vi "GetI.vi"(8 "error in (no error)":errorcluster, 11 "reference in":refnum<class "GOOP4_Sub.lvclass">) -> (0 "error out":errorcluster, 1 "Str 3":string, 2 "i 3":i32, 3 "reference in":refnum<class "GOOP4_Sub.lvclass">)   [LabVIEW 2019, in "GOOP4_Sub.lvclass"]
uses:
  GOOP4_Sub.lvclass
  GOOP4_Base_class/GOOP4_Base.lvclass
  C:/Users/Tiba/Desktop/1GOOP4_CreateObjects_Open_GDS/GOOP4_Base_class/GOOP4_Base.lvclass
panel:
  out "i 2":i32
  out "Str 2":string
  out "Str":string
  out "i":i32
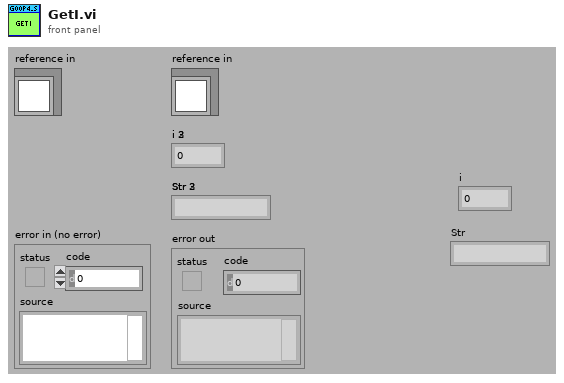
[diagram p1: front panel]
types:
  T1 = typedef "GOOP4_Sub.lvclass/ObjectAttributes.ctl" = cluster{"Str":string, "Boolean":bool}
  T2 = typedef "GOOP4_Base.lvclass/ObjectAttributes.ctl" = cluster{"i":i32}
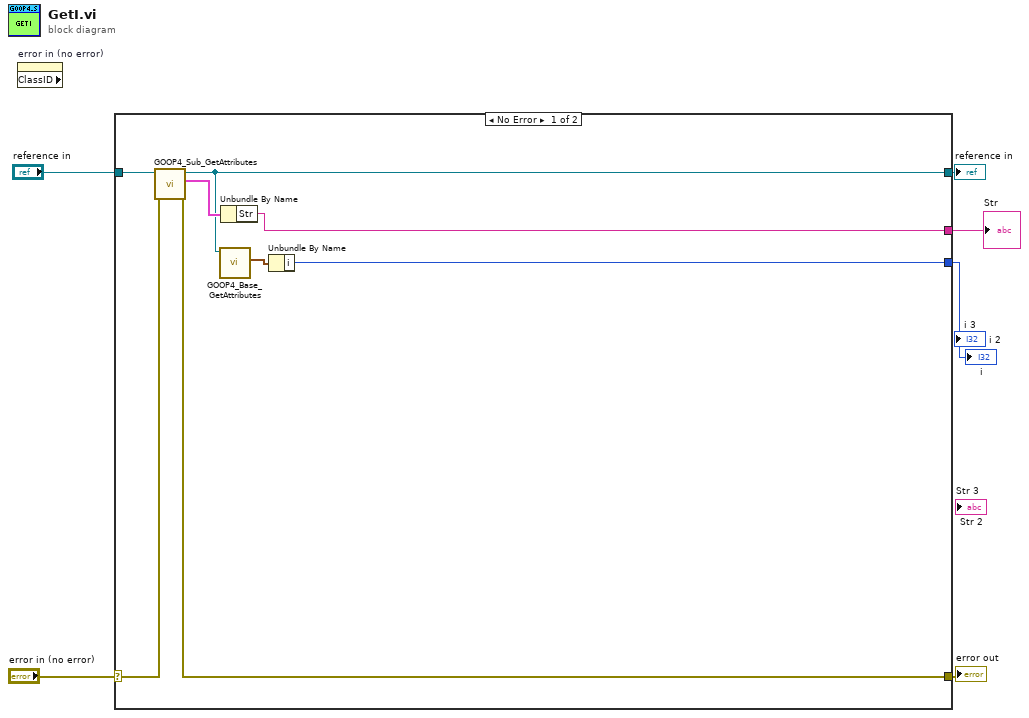
[diagram p0: block diagram]
diagram:
  n1 = property on="error in (no error)" class="Clust (strict)" props=["ClassID"]() -> ()  [unwired: 2 in, 3 out]
  n2 = case shown="No Error" "error in (no error)" {
    selector: "error in (no error)" -> [w14 w16]
    tunnel: [w12 w16] -> w5
    tunnel: [w10 w15] -> w3
    tunnel: "reference in" -> [w11 w15]
    tunnel: [w8 _] -> w2
    tunnel: [w7 _] -> w1
    frame No Error {
      n3 = call "GOOP4_Sub_GetAttributes.vi"("error in (no error)"=w14, "reference in"=w11) -> ("error out"=w12:errorcluster, "Data"=w13:T1, "reference out"=w10:refnum<class "GOOP4_Sub.lvclass">)  [unwired: 6 in, 1 out]
      n4 = call "GOOP4_Base_GetAttributes.vi"("reference in"=w10) -> ("Data"=w9:T2)  [unwired: 7 in, 3 out]
      n5 = Unbundle By Name(w13) -> ("Str"=w7:string)
      n6 = Unbundle By Name(w9) -> ("i"=w8:i32)
    }
    frame Error {
    }
  }
  "error out" <- w5
  "reference in" <- w3
  "i" <- w2
  "Str" <- w1
